vi "RGBtoHSV.vi"(9 "Blue":u8, 10 "Green":u8, 11 "Red":u8) -> (1 "Value":dbl, 2 "Saturation":dbl=1.0, 3 "Hue (0-1)":dbl, 5 "Hue (0-360)":dbl)   [LabVIEW 2014, in "QwaveSys Raspberry Pi Library.lvlib"]
doc: "Convert RGB Values to HSV values. For compatibility with pre-existing HSVtoRGB VI, H is reported in two forms. 0-360 is the \"correct\" format, but other converter uses 0-1 format for H.\n\nH is undefined is S = 0 and will be returned as -1."
uses:
  QwaveSys Raspberry Pi Library.lvlib
panel:
  out "Blue 2":dbl
  out "Green 2":dbl
  out "Red 2":dbl
  # "0-255 Values"
  # "0-1 values"
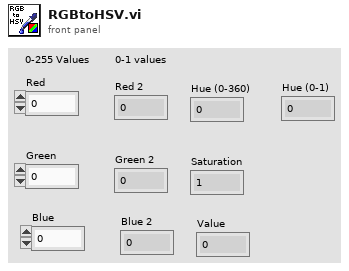
[diagram p1: front panel]
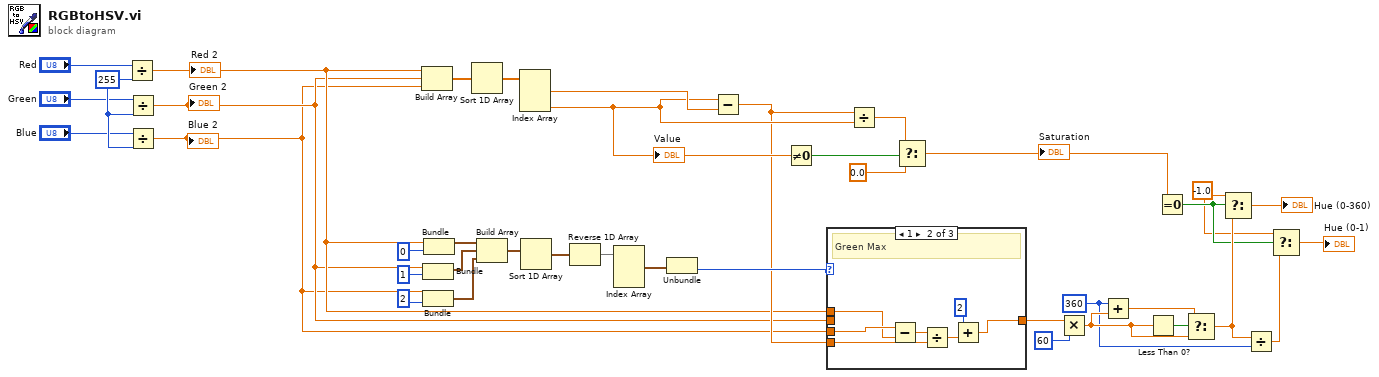
[diagram p0: block diagram]
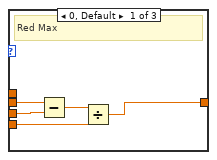
[diagram p2: hidden frame]
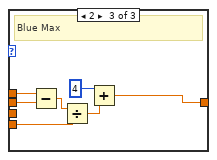
[diagram p3: hidden frame]
diagram:
  w8 = -1.0 ("t")
  w1 = 360
  w22 = 255
  n1 = Divide(x="Red", y=w22) -> (x/y=w19:dbl)
  "Red 2" <- w19
  n2 = Divide(x="Green", y=w22) -> (x/y=w18:dbl)
  "Green 2" <- w18
  n3 = Divide(x="Blue", y=w22) -> (x/y=w17:dbl)
  "Blue 2" <- w17
  n4 = Build Array(w19, w18, w17) -> (w36:dbl[])
  n5 = Bundle(w18, 1) -> (w31:cluster{dbl, i32})  [unwired: 1 in]
  n6 = Bundle(w17, 2) -> (w30:cluster{dbl, i32})  [unwired: 1 in]
  n7 = Bundle(w19, 0) -> (w32:cluster{dbl, i32})  [unwired: 1 in]
  n8 = Sort 1D Array(array=w36) -> (sorted array=w39:dbl[])
  n9 = Build Array(w32, w31, w30) -> (w29:cluster{dbl, i32}[])
  n10 = Index Array(array=w39) -> (element #1=w38:dbl, element #3=w37:dbl)  [unwired: 3 in, 1 out]
  "Value" <- w37
  n11 = Sort 1D Array(array=w29) -> (sorted array=w28:cluster{dbl, i32}[])
  n12 = Reverse 1D Array(array=w28) -> (reversed array=w27:cluster{dbl, i32}[])
  n13 = Index Array(array=w27) -> (element #1=w26:cluster{dbl, i32})  [unwired: 3 in, 2 out]
  n14 = Unbundle(w26) -> (w25:i32)  [unwired: 1 out]
  n15 = Subtract(x=w37, y=w38) -> (x-y=w24:dbl)
  n16 = Not Equal To 0?(x=w37) -> (x != 0?=w7:bool)
  n17 = case shown="1" w25 {
    tunnel: w19 -> [_ w50 w58]
    tunnel: w18 -> [w44 _ w52]
    tunnel: w17 -> [w43 w51 _]
    tunnel: [w40 w45 w53] -> w16
    tunnel: w24 -> [w42 w49 w57]
    frame 0, Default {
      # "Red Max"
      n18 = Subtract(x=w44, y=w43) -> (x-y=w41:dbl)
      n19 = Divide(x=w41, y=w42) -> (x/y=w40:dbl)
    }
    frame 1 {
      # "Green Max"
      n20 = Subtract(x=w51, y=w50) -> (x-y=w48:dbl)
      n21 = Divide(x=w48, y=w49) -> (x/y=w46:dbl)
      n22 = Add(x=2, y=w46) -> (x+y=w45:dbl)
    }
    frame 2 {
      # "Blue Max"
      n23 = Subtract(x=w58, y=w52) -> (x-y=w56:dbl)
      n24 = Divide(x=w56, y=w57) -> (x/y=w54:dbl)
      n25 = Add(x=4, y=w54) -> (x+y=w53:dbl)
    }
  }
  n26 = Divide(x=w24, y=w37) -> (x/y=w5:dbl)
  n27 = Select(t=w5, s=w7, f=0.0) -> (s? t:f=w4:dbl)
  "Saturation" <- w4
  n28 = Multiply(x=w16, y=60) -> (x*y=w3:dbl)
  n29 = Add(x=w1, y=w3) -> (x+y=w14:dbl)
  n30 = Less Than 0?(x=w3) -> (x < 0?=w2:bool)
  n31 = Equal To 0?(x=w4) -> (x = 0?=w11:bool)
  n32 = Select(t=w14, s=w2, f=w3) -> (s? t:f=w12:dbl)
  n33 = Select(t=w8, s=w11, f=w12) -> (s? t:f=→"Hue (0-360)":dbl)
  n34 = Divide(x=w12, y=w1) -> (x/y=w10:dbl)
  n35 = Select(t=w8, s=w11, f=w10) -> (s? t:f=→"Hue (0-1)":dbl)
